vi "2 filtres ds tab historique.vi"(0 "Filtre 1":T1(ring), 1 "valeur recherchée 1":string="MBE", 2 "tab historique":string[][](array[string])=[["112105740008110358\t", "17.03.2008 13:23", "MBE", "9291/07-02.01.01\t", "1", "6"], ["112105740008110259\t", "18.03.2008 13:23", "MBE", "9291/07-02.01.01", "1", "6"], ["112105740008110131\t", "18.03.2008 13:23", "MBE", "9291/07-02.01.01", "1", "6"], ["112105740008110132\t", "18.03.2008 13:23", "MBE", "9291/07-02.01.01", "1", "6"], ["112105740008110255\t", "18.03.2008 13:23", "MBE", "9291/07-02.01.01", "1", "6"], ["112105740008110257\t", "18.03.2008 13:23", "MBE", "9291/07-02.01.01", "1", "6"], ["112105740008090007\t", "03.04.2008 14:12", "MQI", "02692/08-01.01.01", "1", "10"], ["112105740008090006\t", "03.04.2008 14:12", "MQI", "02692/08-01.01.01", "1", "10"], ["112105740008090005", "03.04.2008 14:12", "MQI", "02692/08-01.01.01", "1", "10"], ["112105740008090004\t", "03.04.2008 14:12", "MQI", "02692/08-01.01.01", "1", "10"], ["112105740008090003\t", "03.04.2008 14:12", "MQI", "02692/08-01.01.01", "1", "10"], ["112105740008090002\t", "03.04.2008 14:12", "MQI", "02692/08-01.01.01", "1", "10"], ["112105740008090001", "03.04.2008 14:12", "MQI", "02692/08-01.01.01", "1", "10"]], 3 "Filtre 2":T1(ring)=enum."date", 4 "valeur recherchée 2":string="16.03.2008 13:23") -> (5 "tab pièces correspondantes":string[](array[string]))   [LabVIEW 2011]
panel:
  # "0"
  # "1"
  # "2"
  # "3"
  # "4"
  # "5"
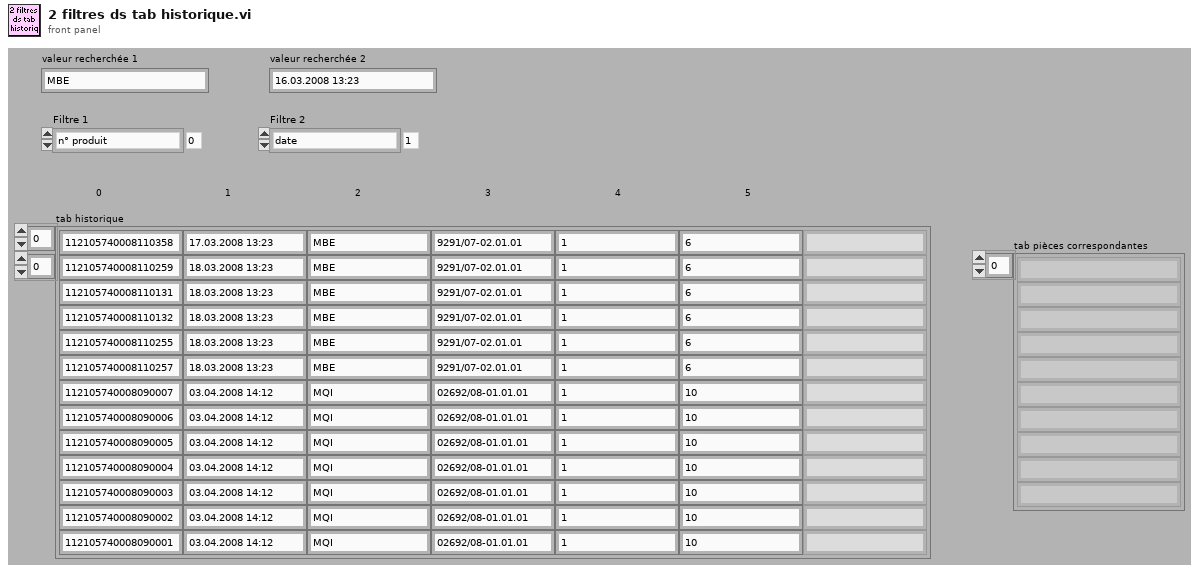
[diagram p1: front panel]
types:
  T1 = enum16{"n° produit", "date", "opérateur", "n° cmde", "n° carton", "qtté cmdée ou retour client"}
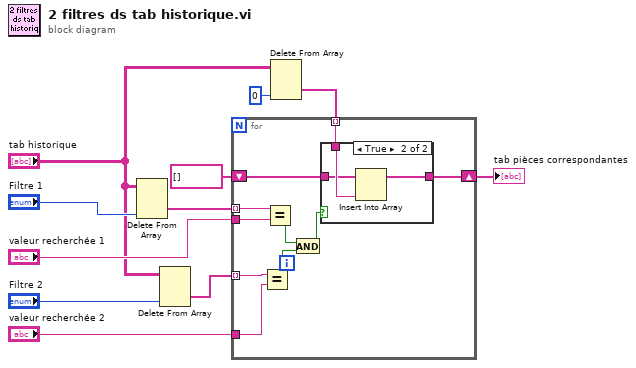
[diagram p0: block diagram]
diagram:
  n1 = Delete From Array(array="tab historique", index (col)="Filtre 1") -> (deleted portion=w11:string[])  [unwired: 2 in, 1 out]
  n2 = Delete From Array(array="tab historique", index (col)="Filtre 2") -> (deleted portion=w1:string[])  [unwired: 2 in, 1 out]
  n3 = Delete From Array(array="tab historique", index (col)=0 ("indice désactivé (col)")) -> (deleted portion=w6:string[])  [unwired: 2 in, 1 out]
  n4 = for {
    tunnel: w11 -> [w20] mode=indexing
    tunnel: "valeur recherchée 1" -> [w21]
    shift-right: [w18] -> w7
    shift-left: string[] [] -> [w17]
    tunnel: w6 -> [w19] mode=indexing
    tunnel: "valeur recherchée 2" -> [w16]
    tunnel: w1 -> [w15] mode=indexing
    n5 = Equal?(x=w15, y=w16) -> (x = y?=w13:bool)
    n6 = Equal?(x=w20, y=w21) -> (x = y?=w14:bool)
    n7 = And(x=w14, y=w13) -> (x .and. y?=w12:bool)
    n8 = case shown="True" w12 {
      tunnel: w19 -> [_ w25]
      tunnel: [w22 w24] -> w18
      tunnel: w17 -> [w22 w23]
      frame False {
      }
      frame True {
        n9 = Insert Into Array(array=w23, new element=w25) -> (w24:string[])  [unwired: 1 in]
      }
    }
  }
  "tab pièces correspondantes" <- w7
